vi "multiplicacion y division.vi"() -> ()   [LabVIEW 2020]
panel:
  out "Waveform Chart":dbl(graph)
  in  "stop":bool
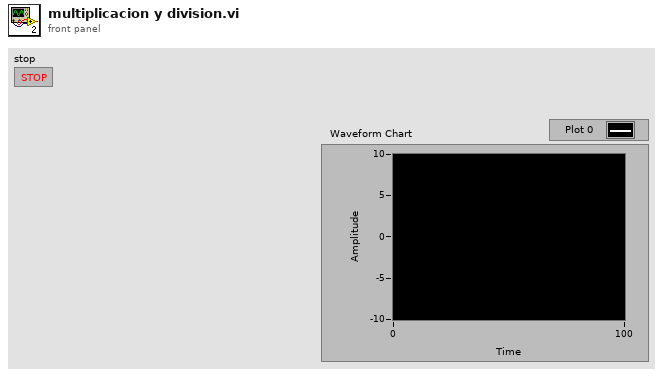
[diagram p1: front panel]
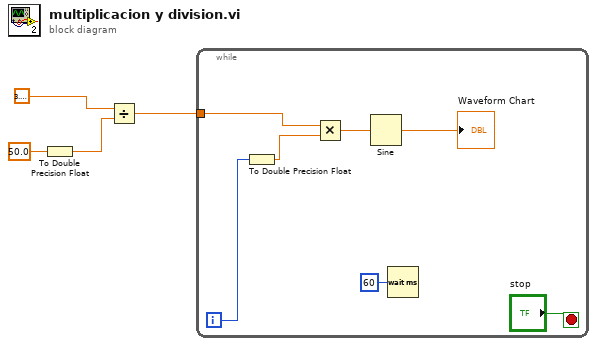
[diagram p0: block diagram]
diagram:
  n1 = To Double Precision Float(number=50.0) -> (double precision float=w3:dbl)
  n2 = Divide(x=3.141592653589793, y=w3) -> (x/y=w4:dbl)
  n3 = while {
    tunnel: w4 -> [w7]
    i -> [w8]
    stop <- "stop" stop-if-true
    n4 = To Double Precision Float(number=w8) -> (double precision float=w9:dbl)
    n5 = Multiply(x=w7, y=w9) -> (x*y=w6:dbl)
    n6 = Sine(x=w6) -> (sin(x)=→"Waveform Chart":dbl)
    n7 = Wait (ms)(milliseconds to wait=u32 60) -> ()  [unwired: 1 out]
  }
